vi "initLicker.vi"(8 "error in (no error)":errorcluster, 10 "Lines":string[](array[string])=["Dev3/ai0", "Dev3/ai1", "Dev3/ai2", "Dev3/ai3", "Dev3/ai4"], 11 "Licker in":refnum<class "Licker.lvclass">) -> (0 "error out":errorcluster, 3 "Licker out":refnum<class "Licker.lvclass">)   [LabVIEW 2014, in "Licker.lvclass"]
uses:
  Licker.lvclass
  Licker.lvclass/Licker.ctl
  <vilib>/DAQmx/create/channels.llb/DAQmx Create Channel (AI-Voltage-Basic).vi
  <vilib>/DAQmx/configure/timing.llb/DAQmx Timing (Sample Clock).vi
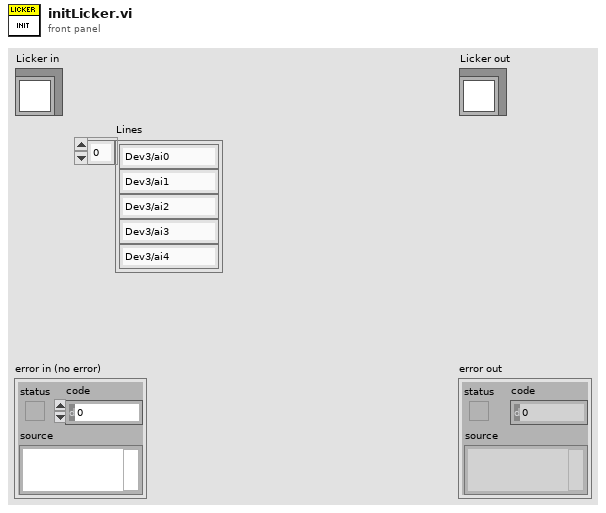
[diagram p1: front panel]
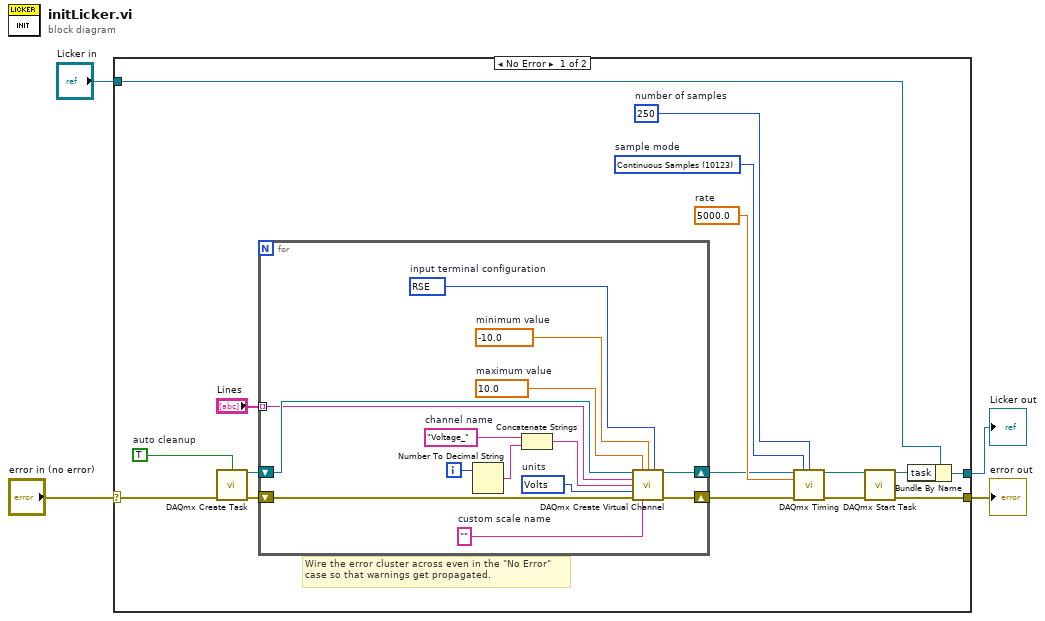
[diagram p0: block diagram]
diagram:
  n1 = case shown="No Error" "error in (no error)" {
    selector: "error in (no error)" -> [w6 w36]
    tunnel: [w18 w36] -> w3
    tunnel: [w19 w35] -> w1
    tunnel: "Licker in" -> [w20 w35]
    frame No Error {
      w13 = 10123 items=["Finite Samples"=10178, "Continuous Samples"=10123, "Hardware Timed Single Point"=12522]  # sample mode
      w14 = 250  # number of samples
      w15 = 5000.0  # rate
      w16 = TRUE  # auto cleanup
      # "Wire the error cluster across even in the \"No Error\"\ncase so that warnings get propagated."
      n2 = call <vilib>:"DAQmx Create Task.vi"("auto cleanup"=w16, "error in"=w6) -> ("task out"=w12:refnum<k21>, "error out"=w11:errorcluster)  [unwired: 12 in]
      n3 = for {
        shift-right: [w30] -> w10
        shift-left: w12 -> [w29]
        shift-right: [w28] -> w9
        shift-left: w11 -> [w27]
        tunnel: "Lines" -> [w21] mode=indexing
        i -> [w25]
        w34 = 10083 items=["default"=-1, "RSE"=10083, "NRSE"=10078, "Differential"=10106, "Pseudodifferential"=12529]  # input terminal configuration
        w33 = 10348 items=["Volts"=10348, "From Custom Scale"=10065]  # units
        w24 = "Voltage_"  # channel name
        w32 = ""  # custom scale name
        w31 = -10.0  # minimum value
        w26 = 10.0  # maximum value
        n4 = Number To Decimal String(number=w25) -> (decimal integer string=w23:string)  [unwired: 1 in]
        n5 = Concatenate Strings(w24, w23) -> (w22:string)
        n6 = call-poly <vilib>:"DAQmx Create Virtual Channel.vi"("task in"=w29, "maximum value"=w26, "minimum value"=w31, "input terminal configuration"=w34, "physical channels"=w21, "name to assign"=w22, "units"=w33, "error in"=w27, "custom scale name"=w32) -> ("task out"=w30:refnum<k21>, "error out"=w28:errorcluster)  [unwired: 5 in]
      }
      n7 = call-poly <vilib>:"DAQmx Timing.vi"("task/channels in"=w10, "sample mode"=w13, "samples per channel"=w14, "rate"=w15, "error in"=w9) -> ("task out"=w8:refnum<k21>, "error out"=w7:errorcluster)  [unwired: 9 in]
      n8 = call <vilib>:"DAQmx Start Task.vi"("task/channels in"=w8, "error in"=w7) -> ("task out"=w17:refnum<k21>, "error out"=w18:errorcluster)  [unwired: 12 in]
      n9 = Bundle By Name(cluster=w20, "task"=w17) -> (w19:refnum<class "Licker.lvclass">)
    }
    frame Error {
    }
  }
  "error out" <- w3
  "Licker out" <- w1
